vi "Tracking Initialization v2.vi"(4 "Eye Model Cluster":T2={"X Grid"=[], "Y Grid"=[], "Za_true Surf"=[], "Iris Center"=[], "Zp_true Surf"=[], "Pinv"=[[1.0, 0.0], [0.0, 1.0]], "za_true"=5.0, "za_work"=1.0, "zp_work"=-1.0, "zp_true"=-5.0}, 5 "Trajectory Cluster":T3, 6 "PID Cluster":T5={"L1 to L4 PID Cluster"={"L1 PID Gains"={"Kp"=0.005, "Kd"=0.5, "Ki"=0.0005}, "L2 PID Gains"={"Kp"=0.01, "Kd"=1.0, "Ki"=0.005}, "L3 PID Gains"={"Kp"=0.05, "Kd"=1.0, "Ki"=0.0005}, "L4 PID Gains"={"Kp"=0.1, "Kd"=0.1, "Ki"=0.0005}}, "Stage PID Cluster"={"Stage Z PID"={"Kp"=0.0005, "Kd"=0.001, "Ki"=0.0}, "Stage Y PID"={"Kp"=0.0003, "Kd"=0.01, "Ki"=0.0}, "Stage X PID"={"Kp"=0.0003, "Kd"=0.01, "Ki"=0.0}}, "OCT Z PID Gains"={"Kp"=0.0003, "Kd"=0.0001, "Ki"=0.01}}, 7 "Robot In":i32, 8 "error in":errorcluster, 9 "Prev Index":i32, 10 "Prev Posit Cluster":T6={"Prev L1 to L4 Posit"=[0.0, 0.0, 0.0, 0.0], "Prev Stage Posit"=[6.0, 6.0, 6.0], "Prev OCT Z Posit"=0.0}, 11 "FPGA VI Reference In":refnum<k20>) -> (0 "error out":errorcluster, 1 "Last Index":i32, 2 "Last Posit Cluster":T4={"Last L1 to L4 Posit"=[0.0, 0.0, 0.0, 0.0], "Last Stage Posit"=[6.0, 6.0, 6.0], "Last OCT Z Posit"=0.0}, 3 "FPGA VI Reference Out":refnum<k20>)   [LabVIEW 2016]
uses:
  Subsystems/Global Variables.vi
  <vilib>/Platform/TimedLoop/XDataNode/wakeup.ctl
  <vilib>/Platform/TimedLoop/XDataNode/XDNodeRunTimeDep.lvlib
  <vilib>/Platform/TimedLoop/XDataNode/nitl_modes.ctl
  <vilib>/Platform/TimedLoop/XDataNode/timing_clust.ctl
  <vilib>/platform/TimedLoop/XDataNode/XDataNode.xnode
  <vilib>/Analysis/Matrix/Datatypes/RealMatrix.ctl
  <vilib>/Analysis/Matrix/NI_Matrix.lvlib
panel:
  out "In Servo Loop":bool
  out "Indexing Finished?":bool
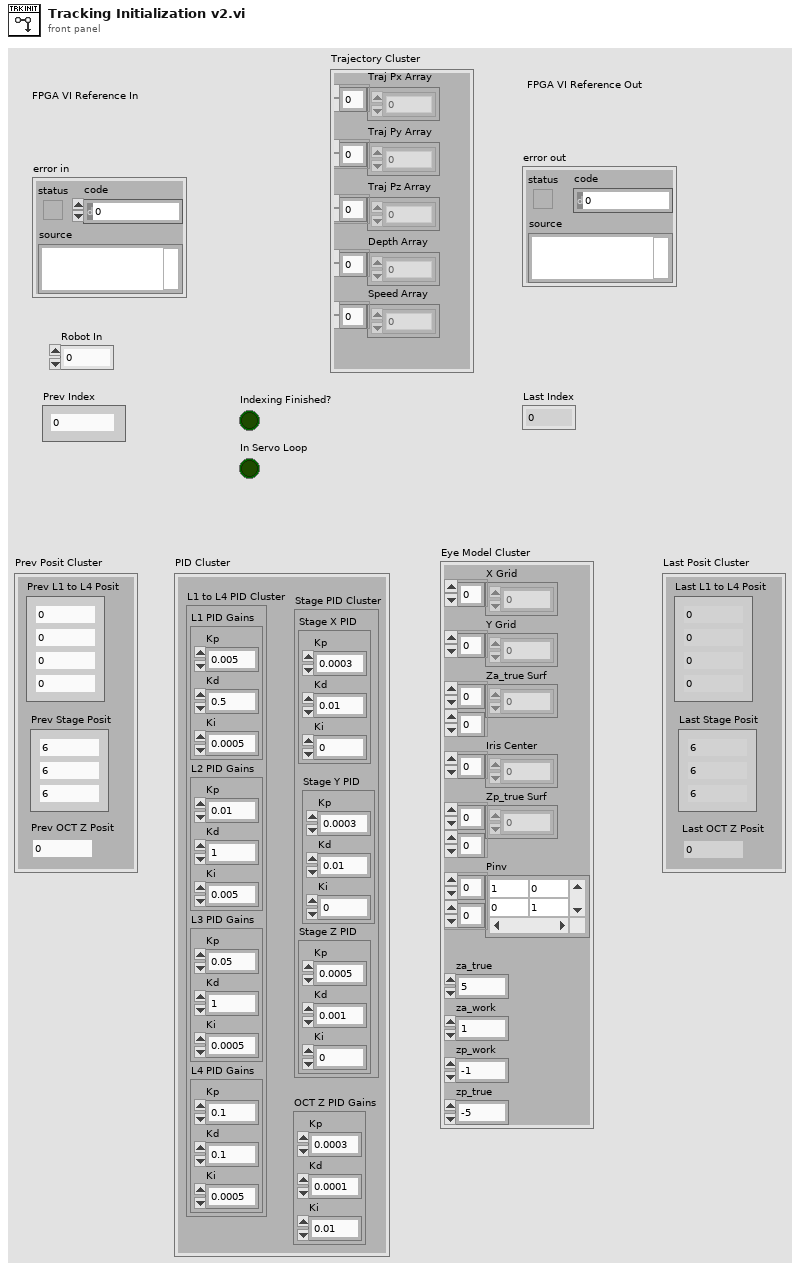
[diagram p1: front panel]
types:
  T1 = typedef "NI_Matrix.lvlib/RealMatrix.ctl" = dbl[][]
  T2 = cluster{"X Grid":dbl[], "Y Grid":dbl[], "Za_true Surf":dbl[][], "Iris Center":dbl[], "Zp_true Surf":dbl[][], "Pinv":T1, "za_true":dbl, "za_work":dbl, "zp_work":dbl, "zp_true":dbl}
  T3 = cluster{"Traj Px Array":dbl[], "Traj Py Array":dbl[], "Traj Pz Array":dbl[], "Speed Array":dbl[], "Depth Array":dbl[]}
  T4 = cluster{"Last L1 to L4 Posit":dbl[], "Last Stage Posit":dbl[], "Last OCT Z Posit":dbl}
  T5 = cluster{"L1 to L4 PID Cluster":cluster{"L1 PID Gains":cluster{"Kp":dbl, "Kd":dbl, "Ki":dbl}, "L2 PID Gains":cluster{"Kp":dbl, "Kd":dbl, "Ki":dbl}, "L3 PID Gains":cluster{"Kp":dbl, "Kd":dbl, "Ki":dbl}, "L4 PID Gains":cluster{"Kp":dbl, "Kd":dbl, "Ki":dbl}}, "Stage PID Cluster":cluster{"Stage Z PID":cluster{"Kp":dbl, "Kd":dbl, "Ki":dbl}, "Stage Y PID":cluster{"Kp":dbl, "Kd":dbl, "Ki":dbl}, "Stage X PID":cluster{"Kp":dbl, "Kd":dbl, "Ki":dbl}}, "OCT Z PID Gains":cluster{"Kp":dbl, "Kd":dbl, "Ki":dbl}}
  T6 = cluster{"Prev L1 to L4 Posit":dbl[], "Prev Stage Posit":dbl[], "Prev OCT Z Posit":dbl}
  T7 = typedef "XDNodeRunTimeDep.lvlib/timing_clust.ctl" = cluster{"Expected End [f-1]":u64, "Actual End [f-1]":u64, "Finished Late? [f-1]":bool, "Expected End [i-1]":u64, "Actual End [i-1]":u64, "Finished Late? [i-1]":bool, "Expected Start [i]":u64, "Actual Start [i]":u64, "Expected Start [f]":u64, "Actual Start [f]":u64, "Source Name":string, "Structure Name":string, "Period":i64, "Deadline":i64, "Offset":i64, "Start":i64, "Priority":i32, "Timeout":i32, "Mode":T8, "Wakeup Reason":T9, "Error":errorcluster, "Source Type":string, "Secondary Source Type":string, "Global End Time":u64, "Global Start Time":u64, "Frame Duration":u64, "Iteration Duration":u64, "Assigned CPU":i32, "I/O Scan Engine Mode":u32}
  T8 = typedef "XDNodeRunTimeDep.lvlib/nitl_modes.ctl" = enum32{"No Change", "Process missed periods, maintain original phase", "Discard missed periods, maintain original phase", "Process missed periods, ignore original phase", "Discard missed periods, ignore original phase"}
  T9 = typedef "XDNodeRunTimeDep.lvlib/wakeup.ctl" = enum32{"Normal", "Aborted", "Asynchronous wakeup", "Timing source error", "Timed loop error", "Timeout"}
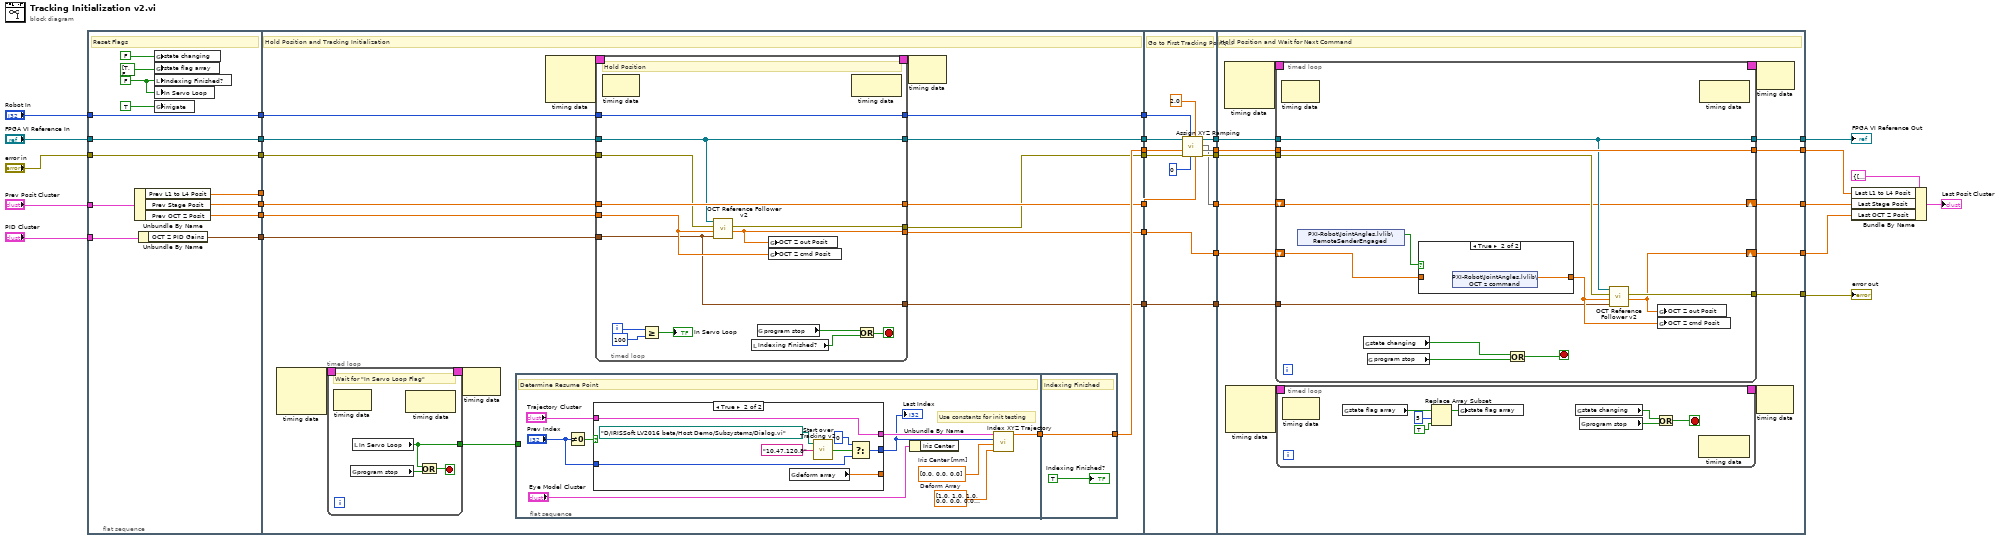
[diagram p0: block diagram]
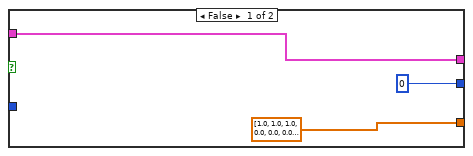
[diagram p2: hidden frame]
diagram:
  n1 = flat-sequence {
    tunnel: [w43] -> w18
    tunnel: "FPGA VI Reference In" -> [w43]
    tunnel: "error in" -> [w42]
    tunnel: [w42] -> w16
    tunnel: [w38] -> w14
    tunnel: "PID Cluster" -> [w37]
    tunnel: "Prev Posit Cluster" -> [w41]
    tunnel: [w40] -> w12
    tunnel: [w39] -> w10
    tunnel: [w35] -> w8
    tunnel: "Robot In" -> [w34]
    tunnel: [w34] -> w2
    tunnel: w18 -> [w62]
    tunnel: [w58] -> w17
    tunnel: w16 -> [w61]
    tunnel: [w48] -> w15
    tunnel: w14 -> [_]
    tunnel: [w57] -> w13
    tunnel: w12 -> [w60]
    tunnel: [w55] -> w11
    tunnel: w10 -> [w59]
    tunnel: [w56] -> w9
    tunnel: w8 -> [w54]
    tunnel: [w53] -> w6
    tunnel: w2 -> [w47]
    tunnel: [w46] -> w1
    tunnel: w17 -> [w122]
    tunnel: w15 -> [w120]
    tunnel: w13 -> [w121]
    tunnel: [w116] -> w31
    tunnel: [w118] -> w30
    tunnel: [w123] -> w27
    tunnel: w11 -> [w113]
    tunnel: [w112] -> w19
    tunnel: w9 -> [w124]
    tunnel: [w124] -> w7
    tunnel: w6 -> [w123]
    tunnel: [w117] -> w4
    tunnel: w1 -> [w115]
    tunnel: [w135] -> w23
    tunnel: w31 -> [w136]
    tunnel: w30 -> [w137]
    tunnel: [w134] -> w28
    tunnel: [w133] -> w29
    tunnel: w27 -> [w132]
    tunnel: [w131] -> w24
    tunnel: [w130] -> w5
    tunnel: w19 -> [w129]
    tunnel: w7 -> [w128]
    tunnel: w4 -> [w127]
    frame #0 {
      w36 = FALSE ("Indexing Finished?")
      # "Reset Flags"
      n2 = Unbundle By Name(w41) -> ("Prev L1 to L4 Posit"=w38:dbl[], "Prev Stage Posit"=w40:dbl[], "Prev OCT Z Posit"=w39:dbl)
      n3 = Unbundle By Name(w37) -> ("OCT Z PID Gains"=w35:cluster{"Kp":dbl, "Kd":dbl, "Ki":dbl})
      n4 = global write "Global Variables.vi" "state changing"(FALSE ("state changing")) -> ()
      n5 = global write "Global Variables.vi" "state flag array"(bool[] [TRUE, FALSE, FALSE, FALSE, FALSE, FALSE, FALSE, FALSE, FALSE] ("state flag array")) -> ()
      n6 = local write "Indexing Finished?"(w36) -> ()
      n7 = local write "In Servo Loop"(w36) -> ()
      n8 = global write "Global Variables.vi" "irrigate"(TRUE ("irrigate")) -> ()
    }
    frame #1 {
      # "Hold Position and Tracking Initialization"
      n9 = node-c288() -> (w52:T7)  [unwired: 3 in]
      n10 = timed-loop {
        timing: w52 -> [_]
        timing-out: [_] -> w51
        tunnel: [w87] -> w50
        stop <- w89 stop-if-true
        # "Wait for \"In Servo Loop Flag\""
        n11 = node-c288() -> ()  [unwired: 1 in, 1 out]
        n12 = global read "Global Variables.vi" "program stop"() -> (w88:bool)
        n13 = local read "In Servo Loop"() -> (w87:bool)
        n14 = node-c288() -> ()  [unwired: 1 in, 1 out]
        n15 = Or(x=w87, y=w88) -> (x .or. y?=w89:bool)
      }
      n16 = node-c288(w51) -> ()  [unwired: 1 out]
      n17 = flat-sequence {
        tunnel: w50 -> [_]
        tunnel: [w65] -> w49
        tunnel: [w85] -> w57
        tunnel: w49 -> [w85]
        frame #0 {
          w66 = dbl[] [1.0, 1.0, 1.0, 0.0, 0.0, 0.0, 0.0, 0.0, 0.0]  # Deform Array
          w67 = dbl[] [0.0, 0.0, 0.0]  # Iris Center [mm]
          # "Use constants for init testing"
          # "Determine Resume Point"
          n18 = Not Equal To 0?(x="Prev Index") -> (x != 0?=w73:bool)
          n19 = case shown="True" w73 {
            tunnel: [0 ("t") w83] -> w68
            tunnel: "Prev Index" -> [_ w82]
            tunnel: "Trajectory Cluster" -> [w75 w81]
            tunnel: [w75 w81] -> w69
            tunnel: [dbl[] [1.0, 1.0, 1.0, 0.0, 0.0, 0.0, 0.0, 0.0, 0.0] ("Deform Array") w80] -> _
            frame False {
            }
            frame True {
              n20 = global read "Global Variables.vi" "deform array"() -> (w80:dbl[])
              n21 = call "Start over Tracking v2.vi"("Host System IP Address"="10.47.120.8", "VI Path on Host"=path "D:/IRISSoft LV2016 beta/Host Demo/Subsystems/Dialog.vi" ("vi path")) -> ("yes/no?"=w79:bool)  [unwired: 2 in, 1 out]
              n22 = Select(t=0, s=w79, f=w82) -> (s? t:f=w83:i32)
            }
          }
          "Last Index" <- w68
          n23 = Unbundle By Name("Eye Model Cluster") -> ()  [unwired: 1 out]
          n24 = call "Index XYZ Trajectory.vi"("Deform Array"=w66, "Pivot Pt"=w67, "Index"=w68, "Trajectory Cluster"=w69) -> ("Indexed XYZ Posit"=w65:dbl[])  [unwired: 6 in, 1 out]
        }
        frame #1 {
          # "Indexing Finished"
          "Indexing Finished?" <- TRUE ("Indexing Finished?")
        }
      }
      n25 = node-c288() -> (w64:T7)  [unwired: 3 in]
      n26 = timed-loop {
        timing: w64 -> [_]
        timing-out: [_] -> w63
        tunnel: w62 -> [w100]
        tunnel: w61 -> [w99]
        tunnel: w60 -> [w101]
        tunnel: w59 -> [w98]
        tunnel: [w100] -> w58
        tunnel: [w97] -> w48
        tunnel: [w101] -> w55
        tunnel: [w96] -> w56
        tunnel: w54 -> [w95]
        tunnel: [w95] -> w53
        tunnel: w47 -> [w94]
        tunnel: [w94] -> w46
        i -> [w104]
        stop <- w106 stop-if-true
        # "Hold Position"
        n27 = node-c288() -> ()  [unwired: 1 in, 1 out]
        n28 = Greater Or Equal?(x=w104, y=100) -> (x >= y?=→"In Servo Loop":bool)
        n29 = call "OCT Reference Follower v2.vi"("OCT Z PID Gains"=w95, "OCT  Z cmd Posit [mm]"=w98, "error in"=w99, "FPGA VI Reference In"=w100) -> ("OCT  Z out Posit [mm]"=w96:dbl, "error out"=w97:errorcluster)  [unwired: 5 in, 1 out]
        n30 = local read "Indexing Finished?"() -> (w105:bool)
        n31 = global read "Global Variables.vi" "program stop"() -> (w107:bool)
        n32 = global write "Global Variables.vi" "OCT Z out Posit"(w96) -> ()
        n33 = global write "Global Variables.vi" "OCT Z cmd Posit"(w98) -> ()
        n34 = node-c288() -> ()  [unwired: 1 in, 1 out]
        n35 = Or(x=w107, y=w105) -> (x .or. y?=w106:bool)
      }
      n36 = node-c288(w63) -> ()  [unwired: 1 out]
    }
    frame #2 {
      # "Go to First Tracking Point/Last Track Point"
      n37 = call "Assign XYZ Ramping.vi"(4:w113, "Ramp Time [sec]"=2.0, "Vac Digital Cmd"=i8 0, "Robot In"=w115, "error in"=w120, "Destination Posit Array [mm]"=w121, "FPGA VI Reference In"=w122) -> ("error out"=w116:errorcluster, 1:w117, 2:w112, "FPGA VI Reference Out"=w118:refnum<k20>)  [unwired: 1 in]
    }
    frame #3 {
      # "Hold Position and Wait for Next Command"
      n38 = node-c288() -> (w139:T7)  [unwired: 3 in]
      n39 = node-c288() -> (w126:T7)  [unwired: 3 in]
      n40 = timed-loop {
        timing: w139 -> [_]
        timing-out: [_] -> w138
        tunnel: w137 -> [w158]
        tunnel: w136 -> [w157]
        tunnel: [w158] -> w135
        tunnel: [w159] -> w134
        tunnel: w132 -> [w153]
        tunnel: [w156] -> w130
        shift-right: [w151] -> w133
        shift-left: w129 -> [w151]
        shift-right: [w155] -> w131
        shift-left: w128 -> [w160]
        tunnel: w127 -> [w159]
        stop <- w161 stop-if-true
        n41 = node-c288() -> ()  [unwired: 1 in, 1 out]
        n42 = shared-variable "PXI-Robot\\JointAngles.lvlib\\RemoteSenderEngaged"() -> (w152:bool)  [unwired: 1 in, 1 out]
        n43 = global read "Global Variables.vi" "state changing"() -> (w163:bool)
        n44 = global read "Global Variables.vi" "program stop"() -> (w162:bool)
        n45 = case shown="True" w152 {
          tunnel: [w164 w165] -> w154
          tunnel: w160 -> [w164 _]
          frame False {
            # "Hold Position if not Engaged"
          }
          frame True {
            n46 = shared-variable "PXI-Robot\\JointAngles.lvlib\\OCT z command"() -> (w165:dbl)  [unwired: 1 in, 1 out]
          }
        }
        n47 = Or(x=w163, y=w162) -> (x .or. y?=w161:bool)
        n48 = call "OCT Reference Follower v2.vi"("OCT Z PID Gains"=w153, "OCT  Z cmd Posit [mm]"=w154, "error in"=w157, "FPGA VI Reference In"=w158) -> ("OCT  Z out Posit [mm]"=w155:dbl, "error out"=w156:errorcluster)  [unwired: 5 in, 1 out]
        n49 = global write "Global Variables.vi" "OCT Z out Posit"(w155) -> ()
        n50 = global write "Global Variables.vi" "OCT Z cmd Posit"(w154) -> ()
        n51 = node-c288() -> ()  [unwired: 1 in, 1 out]
      }
      n52 = timed-loop {
        timing: w126 -> [_]
        timing-out: [_] -> w125
        stop <- w140 stop-if-true
        n53 = node-c288() -> ()  [unwired: 1 in, 1 out]
        n54 = global read "Global Variables.vi" "state flag array"() -> (w145:bool[])
        n55 = Replace Array Subset(array=w145, new element=TRUE ("new element/subarray"), index=5) -> (w144:bool[])
        n56 = global write "Global Variables.vi" "state flag array"(w144) -> ()
        n57 = global read "Global Variables.vi" "state changing"() -> (w146:bool)
        n58 = global read "Global Variables.vi" "program stop"() -> (w141:bool)
        n59 = Or(x=w146, y=w141) -> (x .or. y?=w140:bool)
        n60 = node-c288() -> ()  [unwired: 1 in, 1 out]
      }
      n61 = node-c288(w125) -> ()  [unwired: 1 out]
      n62 = node-c288(w138) -> ()  [unwired: 1 out]
    }
  }
  n63 = Bundle By Name(cluster=T4 {"Last L1 to L4 Posit"=[0.0, 0.0, 0.0, 0.0], "Last Stage Posit"=[6.0, 6.0, 6.0], "Last OCT Z Posit"=0.0} ("Last Posit Cluster 2"), "Last L1 to L4 Posit"=w28, "Last Stage Posit"=w29, "Last OCT Z Posit"=w24) -> (→"Last Posit Cluster":T4)
  "FPGA VI Reference Out" <- w23
  "error out" <- w5
